vi "SendMail.vi"() -> ()   [LabVIEW 2014]
uses:
  <userlib>/Nanonis Prog Interface V5/Nanonis Prog Interface.lvlib
panel:
  out "Emails send":dbl
  in  "stop":bool
  in  "Period [min]":i32
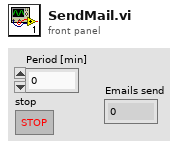
[diagram p1: front panel]
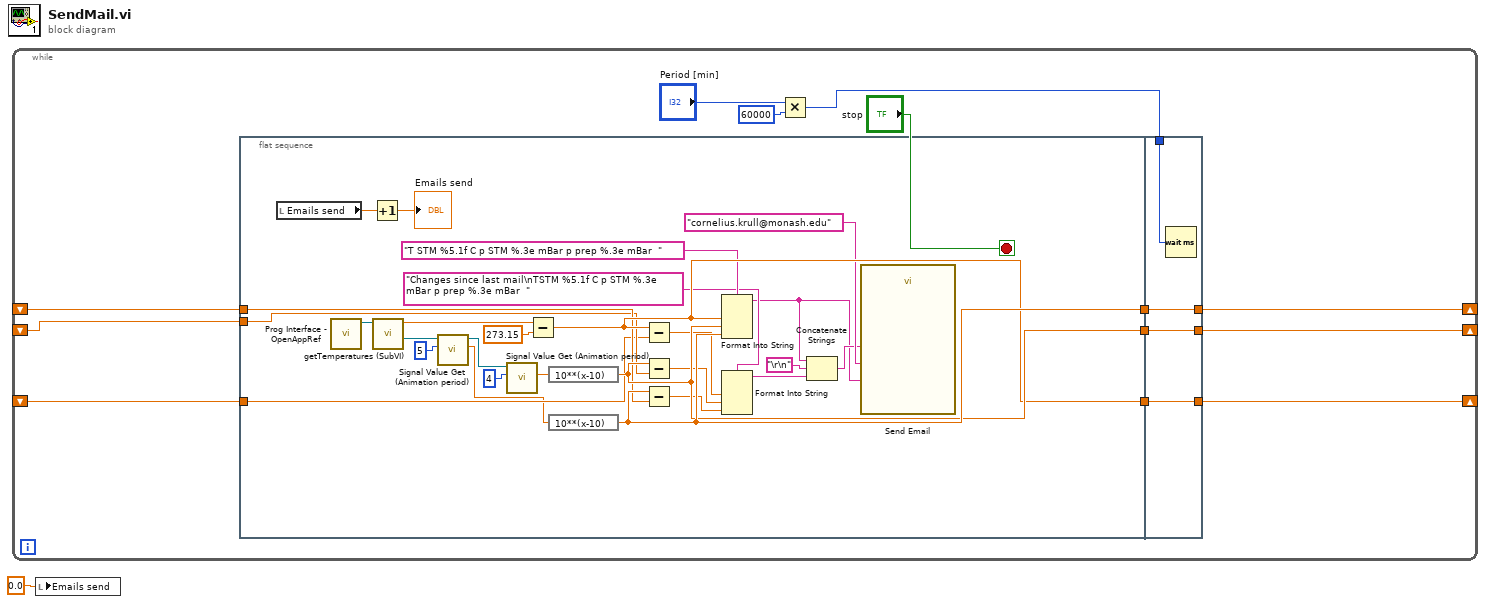
[diagram p0: block diagram]
diagram:
  n1 = while {
    shift-right: [w12] -> _
    shift-left: _ -> [w9]
    shift-right: [w11] -> _
    shift-left: _ -> [w8]
    shift-right: [w10] -> _
    shift-left: _ -> [w7]
    stop <- "stop" stop-if-true
    n2 = flat-sequence {
      tunnel: w9 -> [w38]
      tunnel: w8 -> [w37]
      tunnel: w7 -> [w36]
      tunnel: [w41] -> w5
      tunnel: [w40] -> w4
      tunnel: [w39] -> w3
      tunnel: [w43] -> w10
      tunnel: [w44] -> w11
      tunnel: [w45] -> w12
      tunnel: w5 -> [w45]
      tunnel: w4 -> [w44]
      tunnel: w3 -> [w43]
      tunnel: w2 -> [w42]
      frame #0 {
        n3 = local read "Emails send"() -> (w25:dbl)
        n4 = call <userlib>:"Prog Interface - OpenAppRef.vi"() -> ("Application reference"=w35:refnum<vi>)  [unwired: 6 in, 1 out]
        n5 = Increment(x=w25) -> (x+1=→"Emails send":dbl)
        n6 = call "getTemperatures (SubVI).vi"("Application in"=w35) -> ("Application ref out"=w34:refnum<vi>, "TSTM"=w28:dbl)  [unwired: 7 in, 2 out]
        n7 = call <userlib>:"Signal Value Get (Animation period).vi"("Signal index (0-47)"=i8 5, "Application ref in"=w34) -> ("Signal value"=w30:sgl, "Application ref out"=w33:refnum<vi>)  [unwired: 6 in, 1 out]
        n8 = call <userlib>:"Signal Value Get (Animation period).vi"("Signal index (0-47)"=i8 4, "Application ref in"=w33) -> ("Signal value"=w29:sgl)  [unwired: 6 in, 2 out]
        n9 = Subtract(x=w28, y=273.15) -> (x-y=w39:dbl)
        n10 = expression code="10**(x-10)"(w29) -> (w40:sgl)
        n11 = expression code="10**(x-10)"(w30) -> (w41:sgl)
        n12 = Subtract(x=w39, y=w36) -> (x-y=w19:dbl)
        n13 = Subtract(x=w40, y=w37) -> (x-y=w18:sgl)
        n14 = Subtract(x=w41, y=w38) -> (x-y=w17:sgl)
        n15 = Format Into String(format string="T STM %5.1f C p STM %.3e mBar p prep %.3e mBar  ", w39, w40, w41) -> (resulting string=w15:string)  [unwired: 2 in, 1 out]
        n16 = Format Into String(format string="Changes since last mail\nTSTM %5.1f C p STM %.3e mBar p prep %.3e mBar  ", w19, w18, w17) -> (resulting string=w20:string)  [unwired: 2 in, 1 out]
        n17 = Concatenate Strings(w15, "\r\n", w20) -> (w16:string)
        n18 = call "Send Email"("Message"=w16, "Subject"=w15, "Recipients"="cornelius.krull@monash.edu") -> ()  [unwired: 8 in, 1 out]
      }
      frame #1 {
        n19 = Wait (ms)(milliseconds to wait=w42) -> ()  [unwired: 1 out]
      }
    }
    n20 = Multiply(x="Period [min]", y=60000) -> (x*y=w2:i32)
  }
  n21 = local write "Emails send"(0.0 ("Numeric")) -> ()
